vi "BinaryFormatSaveLoop_dynamicLoad.vi"(8 "data error in":errorcluster, 9 "data queue in":refnum<queue>, 11 "control queue in":refnum<queue>) -> (0 "error out":errorcluster)   [LabVIEW 2013]
uses:
  WriterState.ctl
  Signal_Segment.ctl
  ControlDef/ProcessingMode.ctl
  ControlDef/Files_Format.ctl
  BinaryHeader.ctl
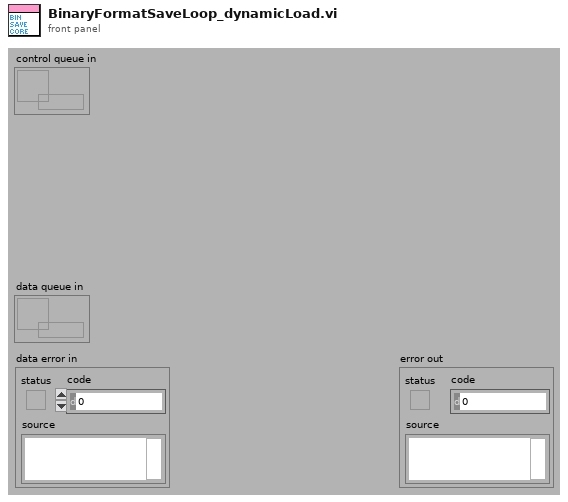
[diagram p1: front panel]
types:
  T1 = enum16{"open", "replace", "create", "open or create", "replace or create", "replace or create with confirmation"}
  T2 = enum16{"big-endian, network order", "native, host order", "little-endian"}
  T3 = typedef "Files_Format.ctl" = enum16{"Text Files", "mzML Files", "Binary Files", "BioMap Files", "imzML Files"}
  T4 = typedef "BinaryHeader.ctl" = cluster{"Start Position":dbl[], "StepWidth":dbl[], "Dimension":i32[], "SpecLength":i32}
  T5 = typedef "WriterState.ctl" = cluster{"State":enum16{"Open", "Close", "ChangeFormat", "SetHeader", "QuitProg."}, "Params":variant}
  T6 = enum16{"Open", "Close", "ChangeFormat", "SetHeader", "QuitProg."}
  T7 = typedef "Signal_Segment.ctl" = cluster{"SampleRate":dbl, "TrigDelay":dbl, "SpecLength":dbl, "DAQ_Range":dbl, "Average#":i32, "Position":dbl[], "Spectrum":sgl[], "Calibr.":dbl[], "Pressure":dbl, "Desp_LaserEnergy":dbl, "PI_LaserEnergy":dbl, "Voltages Table":sgl[][], "ProcMode":T8, "Threshold":dbl, "Comment":string, "TickCount":dbl, "Time Stamp":timestamp}
  T8 = typedef "ProcessingMode.ctl" = enum16{"None", "Drop by Threshold", "TDC Simulate", "SetFilter"}
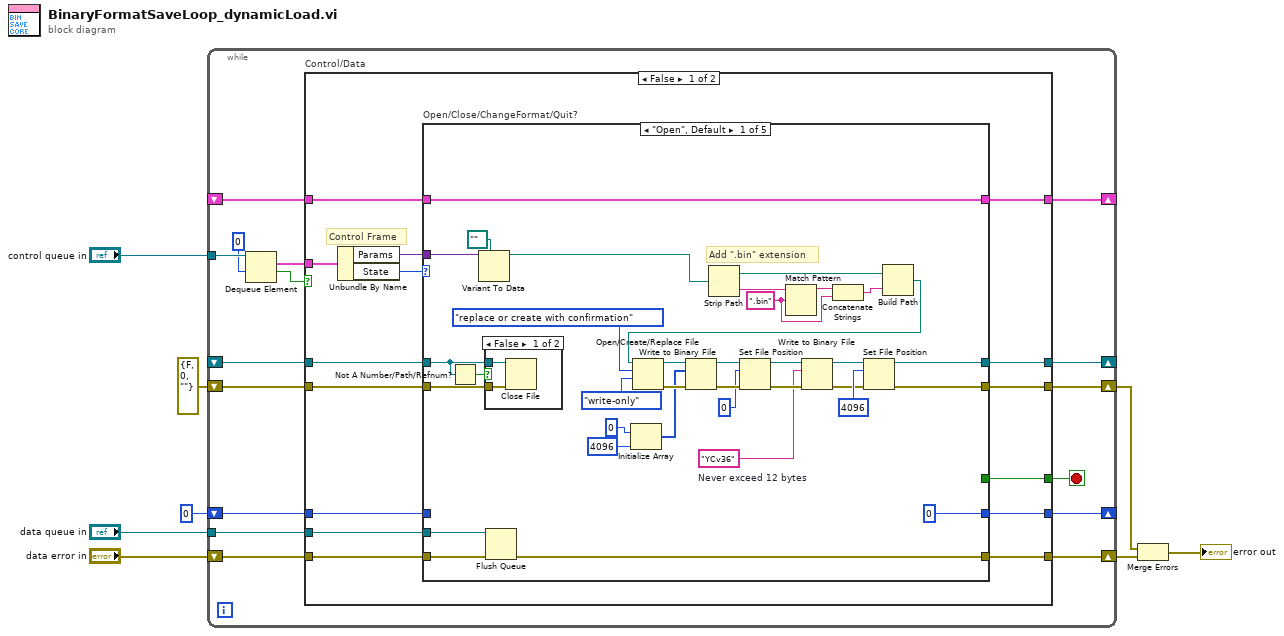
[diagram p0: block diagram]
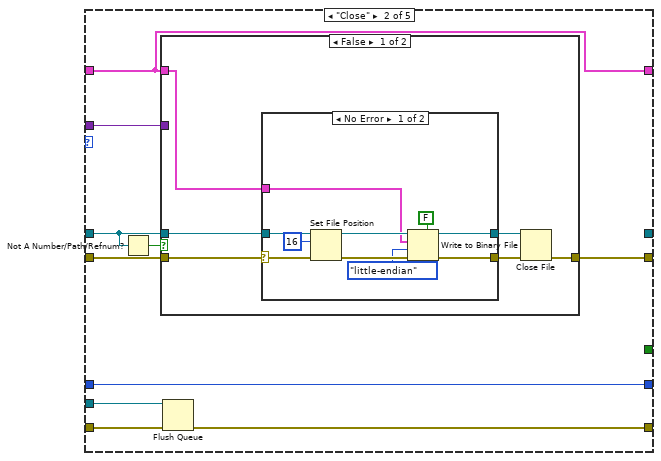
[diagram p3: hidden frame]
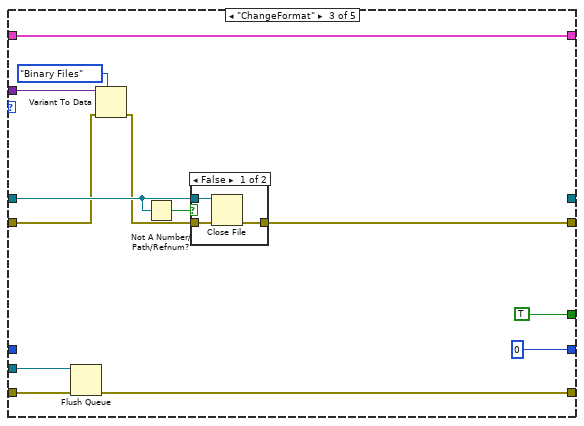
[diagram p6: hidden frame]
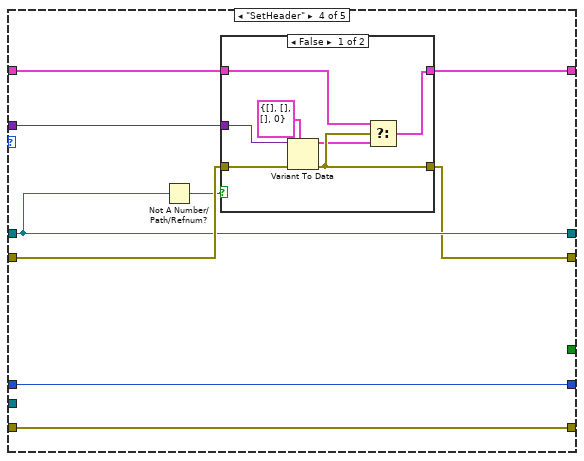
[diagram p8: hidden frame]
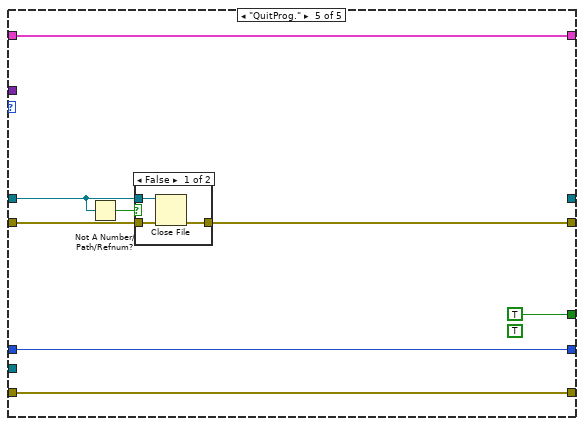
[diagram p10: hidden frame]
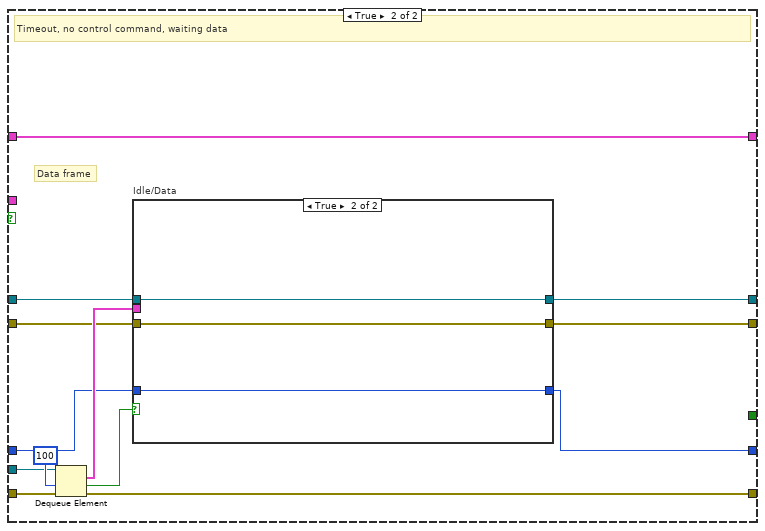
[diagram p12: hidden frame]
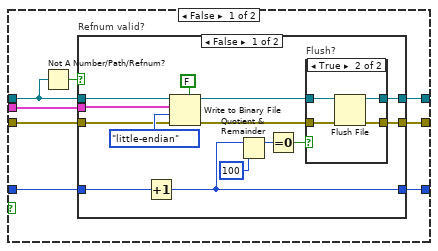
[diagram p13: hidden frame]
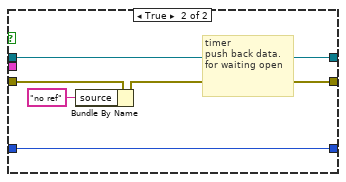
[diagram p15: hidden frame]
diagram:
  n1 = while {
    shift-right: [w19] -> _
    shift-left: 0 -> [w24]
    tunnel: "data queue in" -> [w15]
    shift-right: [w22] -> _
    shift-left: _ -> [w23]
    tunnel: "control queue in" -> [w18]
    shift-right: [w21] -> w1
    shift-left: errorcluster {"status"=FALSE, "code"=0, "source"=""} ("error out") -> [w20]
    shift-right: [w11] -> w8
    shift-left: "data error in" -> [w14]
    shift-right: [w10] -> _
    shift-left: _ -> [w9]
    stop <- w12 stop-if-true
    n2 = Dequeue Element(queue=w18, timeout in ms (-1)=0) -> (element=w13:T5, timed out?=w16:bool)  [unwired: 1 in, 2 out]
    n3 = case "Control/Data" shown="False" w16 {
      tunnel: w24 -> [w30 w157]
      tunnel: w23 -> [w35 w160]
      tunnel: [w34 w159] -> w22
      tunnel: [w33 w158] -> w21
      tunnel: w20 -> [w36 w161]
      tunnel: [w31 w154] -> w19
      tunnel: w15 -> [w28 w164]
      tunnel: w14 -> [w29 w163]
      tunnel: w13 -> [w39 _]
      tunnel: [w32 _] -> w12
      tunnel: [w27 w155] -> w11
      tunnel: [w26 w153] -> w10
      tunnel: w9 -> [w25 w153]
      frame False {
        # "Control Frame"
        n4 = Unbundle By Name(w39) -> ("Params"=w37:variant, "State"=w38:T6)
        n5 = case "Open/Close/ChangeFormat/Quit?" shown="\"Open\", Default" w38 {
          tunnel: w37 -> [w52 w78 w110 w129 _]
          tunnel: w36 -> [w73 w79 w108 w130 w144]
          tunnel: w35 -> [w72 w85 w116 w128 w143]
          tunnel: [w65 _ _ w128 _] -> w34
          tunnel: [w59 w83 w114 w127 w145] -> w33
          tunnel: [_ _ TRUE _ TRUE] -> w32
          tunnel: [0 w84 0 w131 w147] -> w31
          tunnel: w30 -> [_ w84 _ w131 w147]
          tunnel: w29 -> [w68 w82 w112 w123 w142]
          tunnel: w28 -> [w67 w80 w113 _ _]
          tunnel: [w66 w81 w111 w123 w142] -> w27
          tunnel: [w40 w77 w107 w125 w141] -> w26
          tunnel: w25 -> [w40 w77 w107 w126 w141]
          frame "Open", Default {
            w41 = "YCv36"  # Never exceed 12 bytes
            w58 = ".bin" ("regular expression")
            # "Add \".bin\" extension"
            n6 = Not A Number/Path/Refnum?(number/path/refnum=w72) -> (NaN/Path/Refnum?=w74:bool)
            n7 = Variant To Data(type=path "" ("path"), Variant=w52) -> (data=w50:path)  [unwired: 1 in, 1 out]
            n8 = case shown="False" w74 {
              tunnel: w73 -> [w76 _]
              tunnel: w72 -> [w75 _]
              frame False {
                n9 = Close File(refnum=w75, error in=w76) -> ()  [unwired: 2 out]
              }
              frame True {
              }
            }
            n10 = Flush Queue(queue=w67, error in (no error)=w68) -> (error out=w66:errorcluster)  [unwired: 2 out]
            n11 = Initialize Array(u8 0 ("offset (in bytes) (0)"), 4096 ("dimension size")) -> (w47:u8[])
            n12 = Strip Path(path=w50) -> (stripped path=w54:path, name=w55:string)
            n13 = Match Pattern(string=w55, regular expression=w58) -> (before substring=w57:string)  [unwired: 1 in, 3 out]
            n14 = Concatenate Strings(w57, w58) -> (w56:string)
            n15 = Build Path(base path=w54, name or relative path=w56) -> (appended path=w53:path)
            n16 = Open/Create/Replace File(file path (use dialog)=w53, operation (0:open)=T1."replace or create with confirmation", access (0:read/write)=enum16{"read/write", "read-only", "write-only"}."write-only") -> (refnum out=w64:refnum<file>, error out=w60:errorcluster)  [unwired: 3 in, 1 out]
            n17 = Write to Binary File(file (use dialog)=w64, data=w47, error in=w60) -> (refnum out=w43:refnum<file>, error out=w44:errorcluster)  [unwired: 3 in, 1 out]
            n18 = Set File Position(offset (in bytes) (0)=i64 0, refnum=w43, error in=w44) -> (refnum out=w46:refnum<file>, error out=w45:errorcluster)  [unwired: 1 in]
            n19 = Write to Binary File(file (use dialog)=w46, data=w41, error in=w45) -> (refnum out=w48:refnum<file>, error out=w49:errorcluster)  [unwired: 3 in, 1 out]
            n20 = Set File Position(offset (in bytes) (0)=i64 4096, refnum=w48, error in=w49) -> (refnum out=w65:refnum<file>, error out=w59:errorcluster)  [unwired: 1 in]
          }
          frame "Close" {
            n21 = Not A Number/Path/Refnum?(number/path/refnum=w85) -> (NaN/Path/Refnum?=w86:bool)
            n22 = case shown="False" w86 {
              tunnel: w79 -> [w88 w105]
              tunnel: w85 -> [w91 _]
              tunnel: [w92 w105] -> w83
              tunnel: w78 -> [_ _]
              tunnel: w77 -> [w87 _]
              frame False {
                n23 = case shown="No Error" w88 {
                  selector: w88 -> [w97 w103]
                  tunnel: w91 -> [w102 w104]
                  tunnel: [w100 w104] -> w90
                  tunnel: [w99 w103] -> w89
                  tunnel: w87 -> [w93 _]
                  frame No Error {
                    n24 = Set File Position(offset (in bytes) (0)=i64 16, refnum=w102, error in=w97) -> (refnum out=w101:refnum<file>, error out=w98:errorcluster)  [unwired: 1 in]
                    n25 = Write to Binary File(file (use dialog)=w101, data=w93, error in=w98, 5:FALSE ("prepend array or string size? (T)"), 9:T2."little-endian" ("byte order (0:big-endian, network order)")) -> (refnum out=w100:refnum<file>, error out=w99:errorcluster)  [unwired: 1 in, 1 out]
                  }
                  frame Error {
                  }
                }
                n26 = Close File(refnum=w90, error in=w89) -> (error out=w92:errorcluster)  [unwired: 1 out]
              }
              frame True {
              }
            }
            n27 = Flush Queue(queue=w80, error in (no error)=w82) -> (error out=w81:errorcluster)  [unwired: 2 out]
          }
          frame "ChangeFormat" {
            n28 = Flush Queue(queue=w113, error in (no error)=w112) -> (error out=w111:errorcluster)  [unwired: 2 out]
            n29 = Variant To Data(error in=w108, type=Files_Format."Binary Files" ("Format"), Variant=w110) -> (error out=w109:errorcluster)  [unwired: 1 out]
            n30 = Not A Number/Path/Refnum?(number/path/refnum=w116) -> (NaN/Path/Refnum?=w117:bool)
            n31 = case shown="False" w117 {
              tunnel: w109 -> [w121 w122]
              tunnel: w116 -> [w120 _]
              tunnel: [w119 w122] -> w114
              frame False {
                n32 = Close File(refnum=w120, error in=w121) -> (error out=w119:errorcluster)  [unwired: 1 out]
              }
              frame True {
              }
            }
          }
          frame "SetHeader" {
            n33 = Not A Number/Path/Refnum?(number/path/refnum=w128) -> (NaN/Path/Refnum?=w124:bool)
            n34 = case shown="False" w124 {
              tunnel: w130 -> [w138 w139]
              tunnel: w129 -> [w137 _]
              tunnel: [w135 w139] -> w127
              tunnel: w126 -> [w133 w140]
              tunnel: [w132 w140] -> w125
              frame False {
                n35 = Variant To Data(error in=w138, type=T4 {"Start Position"=[], "StepWidth"=[], "Dimension"=[], "SpecLength"=0} ("output cluster"), Variant=w137) -> (data=w134:T4, error out=w135:errorcluster)
                n36 = Select(t=w133, s=w135, f=w134) -> (s? t:f=w132:T4)
              }
              frame True {
              }
            }
          }
          frame "QuitProg." {
            (unwired) TRUE
            n37 = Not A Number/Path/Refnum?(number/path/refnum=w143) -> (NaN/Path/Refnum?=w146:bool)
            n38 = case shown="False" w146 {
              tunnel: w144 -> [w151 w152]
              tunnel: w143 -> [w150 _]
              tunnel: [w149 w152] -> w145
              frame False {
                n39 = Close File(refnum=w150, error in=w151) -> (error out=w149:errorcluster)  [unwired: 1 out]
              }
              frame True {
              }
            }
          }
        }
      }
      frame True {
        # "Data frame"
        # "Timeout, no control command, waiting data"
        n40 = Dequeue Element(queue=w164, timeout in ms (-1)=100, error in (no error)=w163) -> (element=w162:T7, timed out?=w156:bool, error out=w155:errorcluster)  [unwired: 1 out]
        n41 = case "Idle/Data" shown="True" w156 {
          tunnel: w162 -> [w173 _]
          tunnel: w161 -> [w172 w200]
          tunnel: w160 -> [w170 w201]
          tunnel: [w167 w201] -> w159
          tunnel: [w166 w200] -> w158
          tunnel: w157 -> [w169 w199]
          tunnel: [w168 w199] -> w154
          frame False {
            n42 = Not A Number/Path/Refnum?(number/path/refnum=w170) -> (NaN/Path/Refnum?=w171:bool)
            n43 = case "Refnum valid?" shown="False" w171 {
              tunnel: [w175 w196] -> w166
              tunnel: [w176 w198] -> w167
              tunnel: w173 -> [w185 _]
              tunnel: w170 -> [w184 w198]
              tunnel: w172 -> [w183 w197]
              tunnel: w169 -> [w182 w194]
              tunnel: [w179 w194] -> w168
              frame False {
                n44 = Increment(x=w182) -> (x+1=w179:i32)
                n45 = Write to Binary File(file (use dialog)=w184, data=w185, error in=w183, 5:FALSE ("prepend array or string size? (T)"), 9:T2."little-endian" ("byte order (0:big-endian, network order)")) -> (refnum out=w178:refnum<file>, error out=w177:errorcluster)  [unwired: 1 in, 1 out]
                n46 = Quotient & Remainder(x=w179, y=100) -> (x-y*floor(x/y)=w181:i32)  [unwired: 1 out]
                n47 = Equal To 0?(x=w181) -> (x = 0?=w180:bool)
                n48 = case "Flush?" shown="True" w180 {
                  tunnel: w178 -> [w189 w193]
                  tunnel: [w189 w192] -> w176
                  tunnel: w177 -> [w188 w191]
                  tunnel: [w188 w190] -> w175
                  frame False {
                  }
                  frame True {
                    n49 = Flush File(refnum=w193, error in=w191) -> (refnum out=w192:refnum<file>, error out=w190:errorcluster)
                  }
                }
              }
              frame True {
                # "timer\npush back data.\nfor waiting open"
                n50 = Bundle By Name(cluster=w197, "source"="no ref") -> (w196:errorcluster)
              }
            }
          }
          frame True {
          }
        }
      }
    }
  }
  n51 = Merge Errors(w1, w8) -> (→"error out":errorcluster)
